vi "Get Version C.vi"() -> (3 "Version Out":string)   [LabVIEW 2018, in "labview_conan_poc_libc.lvlib"]
uses:
  labview_conan_poc_libc.lvlib
  <vilib>/Utility/LVLibp/NI_PackedLibraryUtility.lvlib
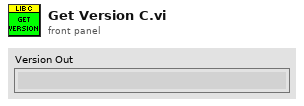
[diagram p1: front panel]
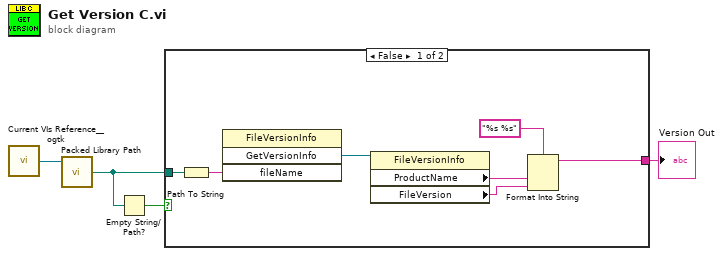
[diagram p0: block diagram]
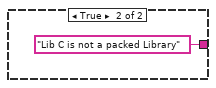
[diagram p2: hidden frame]
diagram:
  n1 = call <userlib>:"Current VIs Reference__ogtk.vi"() -> ("Current VI's reference"=w2:refnum<vi>)  [unwired: 5 in]
  n2 = call <vilib>:"Packed Library Path.vi"("vi reference"=w2) -> ("packed library path"=w4:path)  [unwired: 2 in, 2 out]
  n3 = Empty String/Path?(string/path=w4) -> (empty?=w3:bool)
  n4 = case shown="False" w3 {
    tunnel: w4 -> [w10 _]
    tunnel: [w5 "Lib C is not a packed Library"] -> w1
    frame False {
      n5 = Path To String(path=w10) -> (string=w11:string)
      n6 = invoke class="FileVersionInfo" method="GetVersionInfo"("fileName"=w11) -> ("GetVersionInfo"=w9:refnum<k24>)  [unwired: 3 in, 3 out]
      n7 = property class="FileVersionInfo"(reference=w9) -> ("ProductName"=w7:string, "FileVersion"=w6:string)  [unwired: 1 in, 2 out]
      n8 = Format Into String(format string="%s %s", w7, w6) -> (resulting string=w5:string)  [unwired: 2 in, 1 out]
    }
    frame True {
    }
  }
  "Version Out" <- w1
